vi "AI 1 Samples FPGA（Host）.vi"() -> ()   [LabVIEW 2019]
uses:
  <vilib>/LabVIEW Targets/FPGA/RIO/BlueMoonOnboardIO/nicrio_cRIO-BlueMoonOnboardAi_VoltageRange.ctl
  <vilib>/LabVIEW Targets/FPGA/RIO/BlueMoonOnboardIO/nicrio_cRIO-BlueMoonOnboardAi_TerminalMod.ctl
  <vilib>/FPGAPlugInAG/ELVIS III/niLvFpga_Open_ELVIS III.vi
  <vilib>/rvi/interface/common/dynamic/niFpgaDynamicAddResources.vi
  <vilib>/Utility/error.llb/Error Cluster From Error Code.vi
  <vilib>/rvi/errors/niLvFpgaAdjustHostInterfaceError.vi
  <vilib>/rvi/interface/nirviOpenFPGA/nirviOpenFPGA.xnode
  FPGA Bitfiles/analogio-fpga_FPGATarget_AI1SamplesFPGA_wK2GBALqP+c.lvbitx
  AI 1 Samples FPGA.vi
  <vilib>/rvi/interface/nirviReadWriteControl/nirviReadWriteControl.xnode
  NiFpgaLv.dll
  <vilib>/rvi/interface/Simulation/niFpgaSimulationCallBeginRW.vi
panel:
  out "波形图表":dbl(graph)
  out "数值":dbl
  in  "A?B":bool
  in  "Channel Number":u8
  in  "Terminal Mode":T1=1 items=["DIFF", "RSE"]
  in  "Voltage Range":T2 items=["+/- 10V", "+/- 5V", "+/- 2V", "+/- 1V"]
  in  "采集":bool
  # "结果"
  # "单机时触发"
  # "开始"
  # "配置"
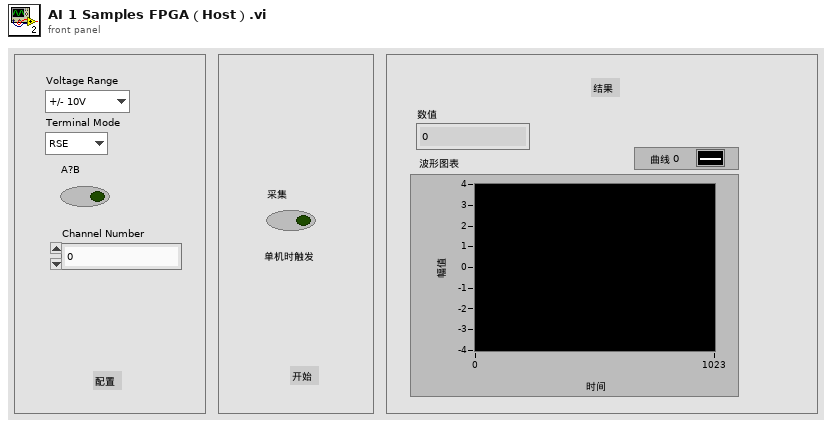
[diagram p1: front panel]
types:
  T1 = typedef "nicrio_cRIO-BlueMoonOnboardAi_TerminalMod.ctl" = u8
  T2 = typedef "nicrio_cRIO-BlueMoonOnboardAi_VoltageRange.ctl" = u8
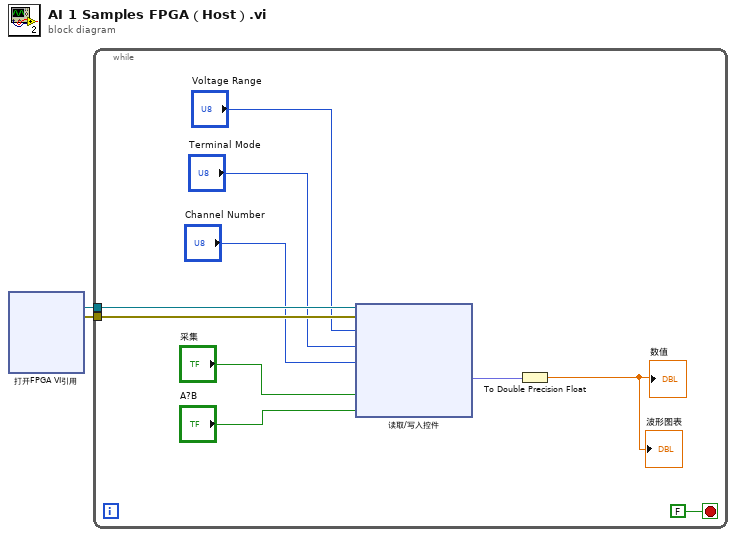
[diagram p0: block diagram]
diagram:
  n1 = xnode "打开FPGA VI引用"() -> ("FPGA VI引用输出"=w2:refnum<k20>, "错误输出"=w1:errorcluster)  [unwired: 2 in]
  n2 = while {
    tunnel: w2 -> [w12]
    tunnel: w1 -> [w11]
    stop <- FALSE stop-if-true
    n3 = xnode "读取/写入控件"("FPGA VI引用输入"=w12, "错误输入"=w11, "Voltage Range"="Voltage Range", "Terminal Mode"="Terminal Mode", "Channel Number"="Channel Number", "Triger Get"="采集", "A?B"="A?B") -> ("Data"=w5:fxp<+/-,24,5>)  [unwired: 2 out]
    n4 = To Double Precision Float(number=w5) -> (double precision float=→"数值" →"波形图表":dbl)
  }
